vi "writetofile.vi"(6 "FilePath":refnum<vi>, 7 "Save Video":bool=TRUE, 8 "error in (no error)":errorcluster, 9 "Rec Flag Reference":refnum<vi>, 10 "Stop Flag Reference":refnum<vi>, 11 "Imaging in":refnum<class "Imaging.lvclass">) -> (0 "error out":errorcluster, 3 "Imaging out":refnum<class "Imaging.lvclass">)   [LabVIEW 2014, in "Imaging.lvclass"]
uses:
  Imaging.lvclass
  Imaging.lvclass/Imaging.ctl
  private/HDF5Tools32/LabView/Append To Dataset 2D Double.vi
  private/HDF5Tools32/LabView/HDF5Tools.lvlib
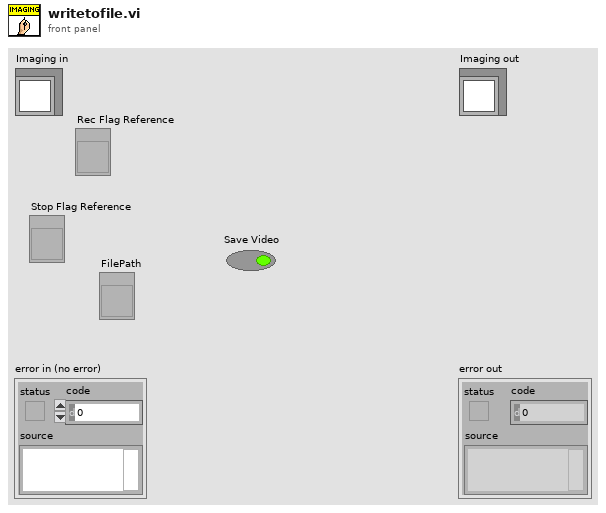
[diagram p1: front panel]
types:
  T1 = typedef "AviRefnum.ctl" = refnum<k1>
  T2 = typedef "IMAQ Image.ctl" = refnum<image>
  T3 = cluster{"Image Out":T2, dbl, "seconds since 1Jan1904":timestamp}
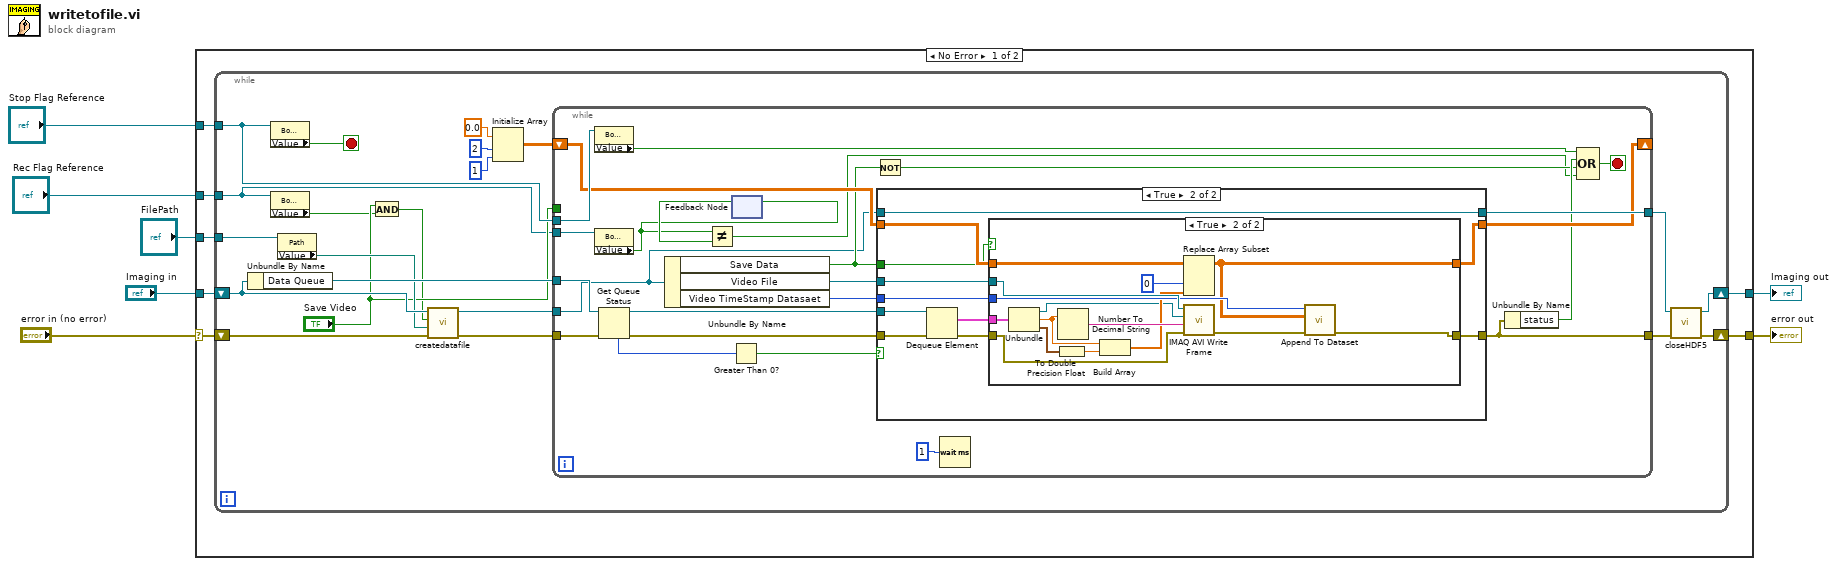
[diagram p0: block diagram]
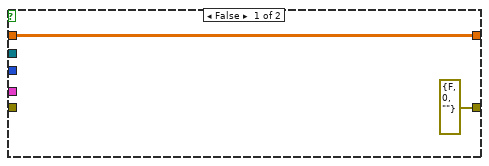
[diagram p3: hidden frame]
diagram:
  n1 = case shown="No Error" "error in (no error)" {
    selector: "error in (no error)" -> [w12 w92]
    tunnel: [w10 w92] -> w6
    tunnel: "Imaging in" -> [w13 w91]
    tunnel: "Stop Flag Reference" -> [w14 _]
    tunnel: [w11 w91] -> w3
    tunnel: "Rec Flag Reference" -> [w9 _]
    tunnel: "FilePath" -> [w8 _]
    frame No Error {
      n2 = while {
        tunnel: w14 -> [w22]
        shift-right: [w24] -> w11
        shift-left: w13 -> [w30]
        shift-right: [w23] -> w10
        shift-left: w12 -> [w28]
        tunnel: w9 -> [w15]
        tunnel: w8 -> [w21]
        stop <- w16 stop-if-true
        n3 = Unbundle By Name(w30) -> ("Data Queue"=w35:refnum<queue>)
        n4 = property class="Bool (strict)"(reference=w22) -> ("Value"=w16:bool)  [unwired: 1 in, 2 out]
        n5 = property class="Bool (strict)"(reference=w15) -> ("Value"=w18:bool)  [unwired: 1 in, 2 out]
        n6 = property class="Path"(reference=w21) -> ("Value"=w20:path)  [unwired: 1 in, 2 out]
        n7 = And(x="Save Video", y=w18) -> (x .and. y?=w17:bool)
        n8 = call-dynamic "createdatafile.vi"("error in (no error)"=w28, "File Path"=w20, "Save Video"=w17, "Imaging in"=w30) -> ("error out"=w27:errorcluster, "Imaging out"=w29:refnum<class "Imaging.lvclass">)  [unwired: 6 in]
        n9 = Initialize Array(0.0 ("element"), 2 ("dimension size"), 1 ("dimension size")) -> (w31:dbl[][])
        n10 = while {
          tunnel: w27 -> [w59]
          tunnel: [w56] -> w25
          tunnel: w22 -> [w57]
          tunnel: w35 -> [w55]
          tunnel: w29 -> [w40]
          tunnel: [w54] -> w26
          shift-right: [w48] -> _
          shift-left: w31 -> [w49]
          tunnel: "Save Video" -> [_]
          tunnel: w15 -> [w39]
          stop <- w45 stop-if-true
          n11 = property class="Bool (strict)"(reference=w57) -> ("Value"=w47:bool)  [unwired: 1 in, 2 out]
          n12 = property class="Bool (strict)"(reference=w39) -> ("Value"=w37:bool)  [unwired: 1 in, 2 out]
          n13 = Get Queue Status(queue=w55, error in (no error)=w59) -> (queue out=w50:refnum<queue>, error out=w58:errorcluster, # elements in queue=w52:i32)  [unwired: 1 in, 5 out]
          n14 = Unbundle By Name(w40) -> ("Save Data"=w43:bool, "Video File"=w42:T1, "Video TimeStamp Datasaet"=w41:i32)
          n15 = Greater Than 0?(x=w52) -> (x > 0?=w53:bool)
          n16 = feedback-in #1(w37) -> ()
          n17 = feedback #1() -> (w38:bool)  [unwired: 1 in]
          n18 = Not Equal?(x=w37, y=w38) -> (x != y?=w36:bool)
          n19 = Not(x=w43) -> (.not. x?=w44:bool)
          n20 = case shown="True" w53 {
            tunnel: w58 -> [w62 w70]
            tunnel: [w62 w68] -> w56
            tunnel: w40 -> [w61 w71]
            tunnel: [w61 w71] -> w54
            tunnel: w50 -> [_ w73]
            tunnel: w49 -> [w60 w67]
            tunnel: [w60 w66] -> w48
            tunnel: w43 -> [_ w65]
            tunnel: w42 -> [_ w64]
            tunnel: w41 -> [_ w63]
            frame False {
            }
            frame True {
              n21 = Dequeue Element(queue=w73, error in (no error)=w70) -> (element=w72:T3, error out=w69:errorcluster)  [unwired: 1 in, 2 out]
              n22 = case shown="True" w65 {
                tunnel: [errorcluster {"status"=FALSE, "code"=0, "source"=""} ("Error out") w84] -> w68
                tunnel: w72 -> [_ w90]
                tunnel: w64 -> [_ w87]
                tunnel: w63 -> [_ w86]
                tunnel: w69 -> [_ w78]
                tunnel: w67 -> [w74 w81]
                tunnel: [w74 w79] -> w66
                frame False {
                }
                frame True {
                  n23 = Unbundle(w90) -> ("Image Out"=w77:T2, w88:dbl, "seconds since 1Jan1904"=w82:timestamp)
                  n24 = To Double Precision Float(number=w82) -> (double precision float=w83:dbl)
                  n25 = Number To Decimal String(number=w88) -> (decimal integer string=w89:string)  [unwired: 1 in]
                  n26 = Build Array(w88, w83) -> (w80:dbl[])
                  n27 = Replace Array Subset(array=w81, new element=w80, index (col)=0 ("disabled index (col)")) -> (w79:dbl[][])  [unwired: 1 in]
                  n28 = call "IMAQ AVI Write Frame"("error in (no error)"=w78, "Data"=w89, "Image"=w77, "Avi Refnum"=w87) -> ("error out"=w85:errorcluster)  [unwired: 7 out]
                  n29 = call-poly "Append To Dataset.vi"("Error in (no error)"=w85, "Data"=w79, "Dataset id in"=w86) -> ("Error out"=w84:errorcluster)  [unwired: 7 in, 1 out]
                }
              }
            }
          }
          n30 = Wait (ms)(milliseconds to wait=u32 1) -> ()  [unwired: 1 out]
          n31 = Unbundle By Name(w56) -> ("status"=w46:bool)
          n32 = Compound Arithmetic op=OR(w47, w46, w44, w36) -> (w45:bool)
        }
        n33 = call-dynamic "closeHDF5.vi"("error in (no error)"=w25, "Imaging in"=w26) -> ("error out"=w23:errorcluster, "Imaging out"=w24:refnum<class "Imaging.lvclass">)  [unwired: 8 in]
      }
    }
    frame Error {
    }
  }
  "error out" <- w6
  "Imaging out" <- w3
